vi "Upload Part.vi"(8 "error in (no error)":errorcluster, 9 "Part Number":i32=1, 10 "Data":string, 11 "Multipart Upload in":refnum<class "Multipart Upload.lvclass">) -> (0 "error out":errorcluster, 3 "Multipart Upload out":refnum<class "Multipart Upload.lvclass">)   [LabVIEW 2015, in "NI_AWS_S3.lvlib" / "Multipart Upload.lvclass"]
uses:
  Multipart Upload.lvclass
  Core/HTTP Request/Name Value Pair.ctl
  Core/HTTP Request/Request Options.ctl
  Core/HTTP Request/Region handling.ctl
  Core/HTTP Request/URL formatting.ctl
  Part.ctl
  Multipart Upload.lvclass/Multipart Upload.ctl
  Bucket/Bucket.lvclass/Bucket.ctl
  Read Bucket.vi
  Read Parts.vi
  Read Upload ID.vi
  Read Object Key.vi
  Bucket/Read Name.vi
  Write Bucket.vi
  Write Parts.vi
  Bucket/Bucket.lvclass
  Core/HTTP Request/HTTP Request.lvclass
  NI_AWS_S3.lvlib
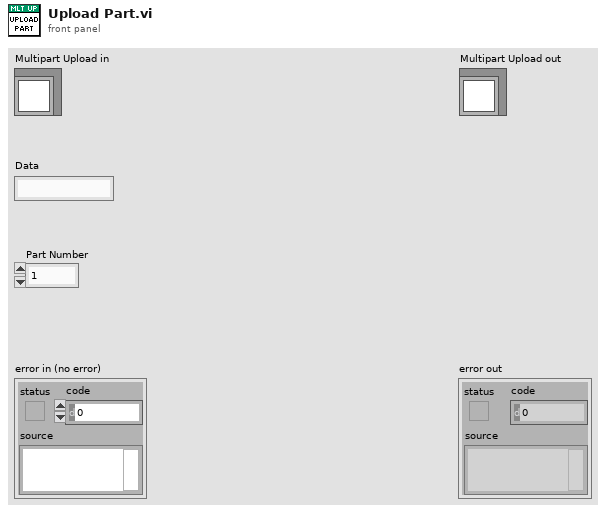
[diagram p1: front panel]
types:
  T1 = typedef "NI_AWS_S3.lvlib/Part.ctl" = cluster{"Part Number":i32, "Last Modified":timestamp, "ETag":string, "Size":i32}
  T2 = typedef "NI_AWS_Core.lvlib/HTTP Request.lvclass/Region handling.ctl" = enum16{"use region everywhere", "use region (authentication only)", "use region (URL only)", "ignore region everwhere"}
  T3 = typedef "NI_AWS_Core.lvlib/HTTP Request.lvclass/Request Options.ctl" = cluster{"request headers":T4[], "request parameters":T4[], "request body":string, "region handling":T2, "URL formatting":T5}
  T4 = typedef "NI_AWS_Core.lvlib/HTTP Request.lvclass/Name Value Pair.ctl" = cluster{"name":string, "value":string}
  T5 = typedef "NI_AWS_Core.lvlib/HTTP Request.lvclass/URL formatting.ctl" = enum16{"region-", "region."}
  T6 = typedef "NI_AWS_Core.lvlib/HTTP Request.lvclass/Response.ctl" = cluster{"Headers":string, "Body":string}
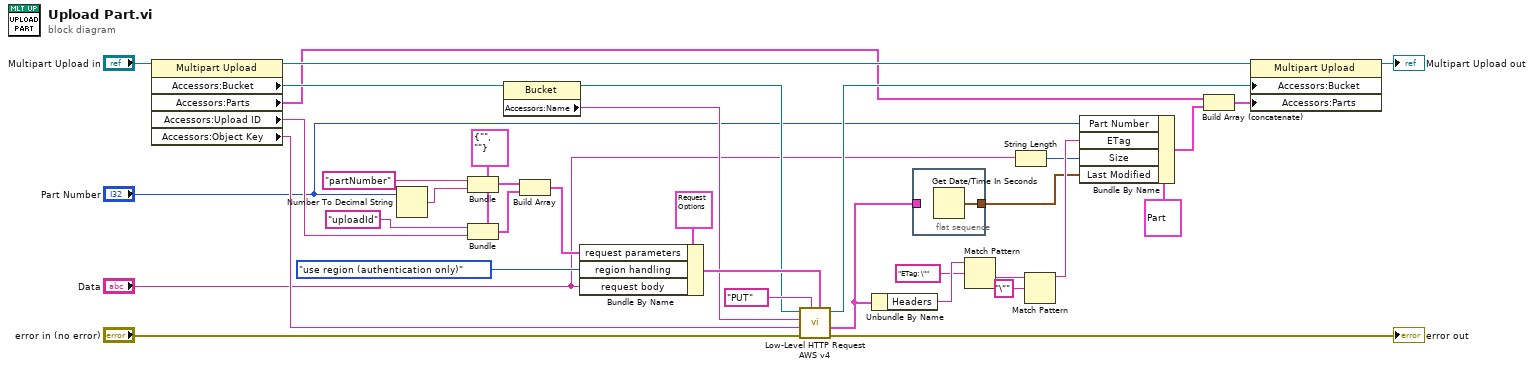
[diagram p0: block diagram]
diagram:
  w30 = T4 {"name"="", "value"=""} ("Name Value Pair")
  n1 = property class="Multipart Upload"(reference="Multipart Upload in") -> (reference out=w23:refnum<class "Multipart Upload.lvclass">, "Accessors:Bucket"=w24:refnum<class "Bucket.lvclass">, "Accessors:Parts"=w14:T1[], "Accessors:Upload ID"=w15:string, "Accessors:Object Key"=w18:string)  [unwired: 1 in, 1 out]
  n2 = Number To Decimal String(number="Part Number") -> (decimal integer string=w34:string)  [unwired: 1 in]
  n3 = Bundle(cluster=w30, "name"="partNumber" ("format string"), "value"=w34) -> (w33:T4)
  n4 = Bundle(cluster=w30, "name"="uploadId" ("format string"), "value"=w15) -> (w32:T4)
  n5 = property class="Bucket"(reference=w24) -> (reference out=w20:refnum<class "Bucket.lvclass">, "Accessors:Name"=w19:string)  [unwired: 1 in, 1 out]
  n6 = Build Array(w33, w32) -> (w16:T4[])
  n7 = Bundle By Name(cluster=T3 {"request headers"=[], "request parameters"=[], "request body"="", "region handling"=enum."use region everywhere", "URL formatting"=enum."region."} ("Request Options"), "request parameters"=w16, "region handling"=Region_handling."use region (authentication only)", "request body"="Data") -> (w28:T3)
  n8 = call "Low-Level HTTP Request AWS v4.vi"("Request Options"=w28, "HTTP-Verb"="PUT", "error in (no error)"="error in (no error)", "URL Suffix"=w18, "URL Prefix"=w19, "AWS Core in"=w20) -> ("error out"=→"error out":errorcluster, "Response"=w1:T6, "AWS Core out"=w21:refnum<class "Bucket.lvclass">)  [unwired: 2 in, 1 out]
  n9 = Unbundle By Name(w1) -> ("Headers"=w9:string)
  n10 = flat-sequence {
    tunnel: [w37] -> w2
    tunnel: w1 -> [_]
    frame #0 {
      n11 = Get Date/Time In Seconds() -> (seconds since 1Jan1904=w37:timestamp)
    }
  }
  n12 = Match Pattern(string=w9, regular expression="ETag: \"") -> (after substring=w7:string)  [unwired: 1 in, 3 out]
  n13 = String Length(string="Data") -> (length=w4:i32)
  n14 = Match Pattern(string=w7, regular expression="\"") -> (before substring=w5:string)  [unwired: 1 in, 3 out]
  n15 = Bundle By Name(cluster=T1 {"Part Number"=0, "Last Modified"=timestamp(0 s since 1904-01-01), "ETag"="", "Size"=0} ("Part"), "Part Number"="Part Number", "ETag"=w5, "Size"=w4, "Last Modified"=w2) -> (w11:T1)
  n16 = Build Array (concatenate)(w14, w11) -> (w13:T1[])
  n17 = property class="Multipart Upload"(reference=w23, "Accessors:Bucket"=w21, "Accessors:Parts"=w13) -> (reference out=→"Multipart Upload out":refnum<class "Multipart Upload.lvclass">)  [unwired: 1 in, 1 out]
